vi "TEST Object Manual Bounds (Non Default Scaling).vi"() -> ()   [LabVIEW 2021, in "IObject.lvclass"]
uses:
  IObject.lvclass
  <vilib>/Utility/miscctls.llb/LVRectTypeDef.ctl
  Object/Object.lvclass
panel:
  in  "Bounds":T1={"Left"=100, "Top"=50, "Right"=200, "Bottom"=150}
  in  "OK Button":bool
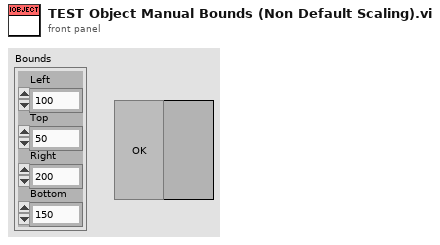
[diagram p1: front panel]
types:
  T1 = typedef "LVRectTypeDef.ctl" = cluster{"Left":i16, "Top":i16, "Right":i16, "Bottom":i16}
  T2 = cluster{"Left":dbl, "Top":dbl, "Right":dbl, "Bottom":dbl}
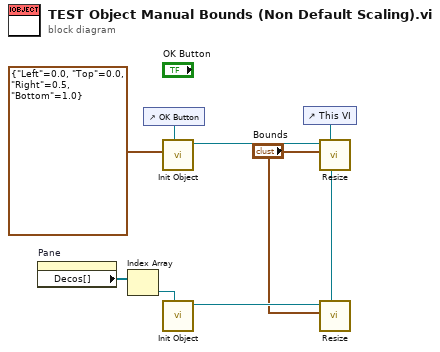
[diagram p0: block diagram]
diagram:
  n1 = property on="Pane" class="Pane"() -> ("Decos[]"=w6:refnum<vi>[])  [unwired: 2 in, 2 out]
  n2 = Index Array(array=w6) -> (element=w4:refnum<vi>)  [unwired: 1 in]
  n3 = control-ref of="OK Button"() -> (w8:refnum<vi>)
  n4 = call "Init Object.vi"("GObj Refnum"=w8, "A [0, 0, 1, 1]"=T2 {"Left"=0.0, "Top"=0.0, "Right"=0.5, "Bottom"=1.0}) -> ("MMI Scaling out"=w7:refnum<class "Object.lvclass">)  [unwired: 8 in, 1 out]
  n5 = call "Init Object.vi"("GObj Refnum"=w4) -> ("MMI Scaling out"=w5:refnum<class "Object.lvclass">)  [unwired: 9 in, 1 out]
  n6 = control-ref of="This VI"() -> (w3:refnum<vi>)
  n7 = call-dynamic "Resize.vi"("VI Refnum"=w3, "Bounds"="Bounds", "MMI Scaling in"=w7) -> ()  [unwired: 6 in, 3 out]
  n8 = call-dynamic "Resize.vi"("VI Refnum"=w3, "Bounds"="Bounds", "MMI Scaling in"=w5) -> ()  [unwired: 6 in, 3 out]
